vi "setDataRetrievalMethod.vi"(0 "CCD in":refnum<class "CCD.lvclass">, 5 "error in (no error)":errorcluster) -> (14 "CCD out":refnum<class "CCD.lvclass">, 15 "results-JSON string":string, 16 "ID":i32, 17 "returned command":string, 18 "error string (if existing)":string, 19 "error out":errorcluster)   [LabVIEW 2023, in "CCD.lvclass"]
uses:
  CCD.lvclass
  20f7d3bd-08ac-4524-9bed-df36c1da25a0.vi
  <vilib>/JDP Science/JSONtext/Variant to JSON Text.vi
  <vilib>/JDP Science/JSONtext/Set Item.vi
  <vilib>/JDP Science/JSONtext/LVClass Serializer/JSONtext LVClass Serializer.lvclass
  CCD.lvclass/CCD.ctl
  GenericDevice/GenericDevice.lvclass
panel:
  # "Connector Pane"
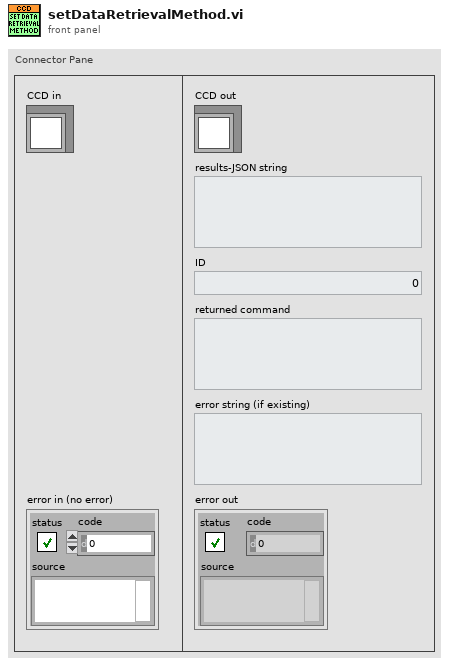
[diagram p1: front panel]
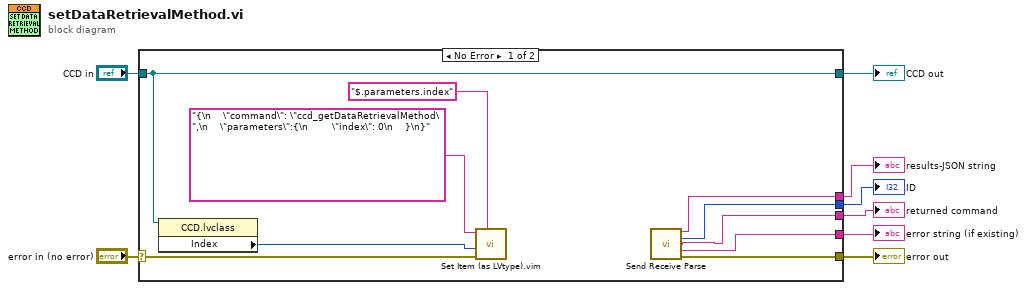
[diagram p0: block diagram]
diagram:
  n1 = case shown="No Error" "error in (no error)" {
    selector: "error in (no error)" -> [w15 w21]
    tunnel: [w14 w21] -> w7
    tunnel: [w17 w20] -> w5
    tunnel: "CCD in" -> [w17 w20]
    tunnel: [w13 _] -> w4
    tunnel: [w12 _] -> w3
    tunnel: [w11 _] -> w2
    tunnel: [w10 _] -> w1
    frame No Error {
      n2 = property class="CCD.lvclass"(reference=w17) -> ("Index"=w16:i32)  [unwired: 1 in, 2 out]
      n3 = call "Set Item (as LVtype).vim"("$Path or Item Name"="$.parameters.index", "error in (no error)"=w15, "Anything"=w16, "JSON"="{\n    \"command\": \"ccd_getDataRetrievalMethod\",\n    \"parameters\":{\n        \"index\": 0\n    }\n}") -> ()  [unwired: 4 in, 3 out]
      n4 = call "Send Receive Parse.vi"() -> ("<JSON>"=w9:string, "results-JSON string"=w13:string, "ID"=w12:i32, "returned command"=w11:string, "error string (if existing)"=w10:string, "error out"=w14:errorcluster)  [unwired: 10 in]
    }
    frame Error {
    }
  }
  "error out" <- w7
  "CCD out" <- w5
  "results-JSON string" <- w4
  "ID" <- w3
  "returned command" <- w2
  "error string (if existing)" <- w1
